vi "Set Status.vi"(6 "Status Message":string, 7 "Action":enum16{"Set Ref", "Set Message"}(ring)=enum."Set Message", 8 "error in (no error)":errorcluster, 11 "Status Ref":refnum<vi>) -> (0 "error out":errorcluster)   [LabVIEW 2023]
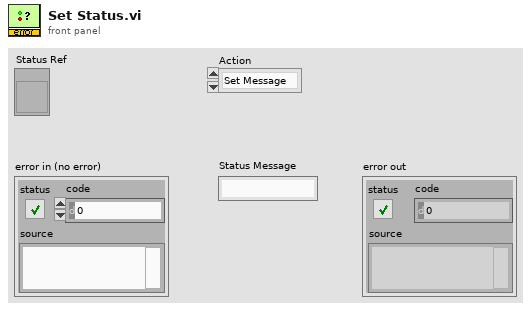
[diagram p1: front panel]
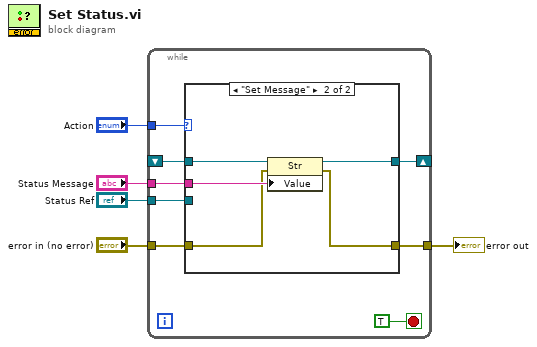
[diagram p0: block diagram]
diagram:
  n1 = while {
    tunnel: "Action" -> [w13]
    shift-right: [w12] -> _
    shift-left: _ -> [w10]
    tunnel: "Status Ref" -> [w11]
    tunnel: "Status Message" -> [w9]
    tunnel: "error in (no error)" -> [w8]
    tunnel: [w7] -> w1
    stop <- TRUE stop-if-true
    n2 = case shown="\"Set Message\"" w13 {
      tunnel: [w15 w19] -> w12
      tunnel: w11 -> [w15 _]
      tunnel: w10 -> [_ w20]
      tunnel: w9 -> [_ w18]
      tunnel: w8 -> [w14 w17]
      tunnel: [w14 w16] -> w7
      frame "Set Ref", Default {
      }
      frame "Set Message" {
        n3 = property class="Str"(reference=w20, error in=w17, "Value"=w18) -> (reference out=w19:refnum<vi>, error out=w16:errorcluster)
      }
    }
  }
  "error out" <- w1
